vi "CalcPixelShifts.vi"(0 "Sampling Rate (Hz)":dbl=1000000000.0, 1 "c (m/s)":i16=1485, 2 "delay (mm)":sgl, 3 "rf pts":i32, 5 "ROC (m)":dbl=0.012, 9 "Radii (m)":sgl[](array[numeric])=[0.0, 0.00132, 0.00142, 0.0019, 0.002, 0.00236, 0.00245, 0.00275, 0.00285, 0.0031], 11 "One Way Receive":bool, 14 "Dual mode":bool) -> (15 "InterpIndex":sgl[][](array[numeric]))   [LabVIEW 2022 SP3]
panel:
  out "z grid RF samps":dbl[](array[numeric])
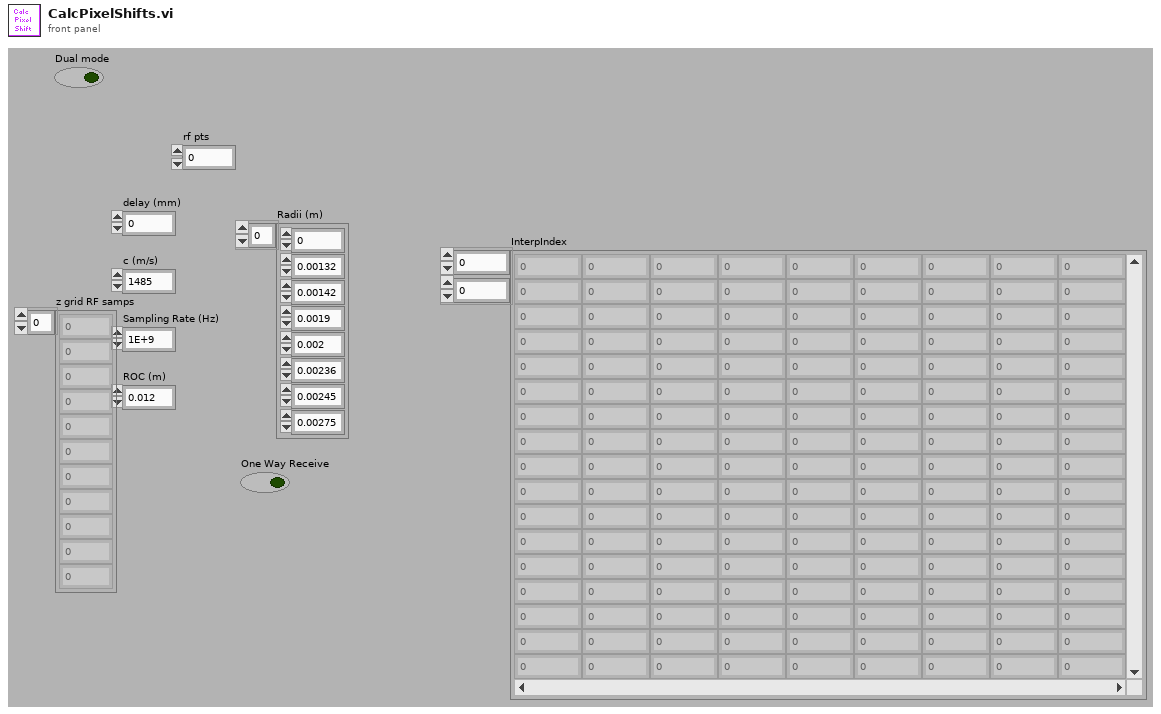
[diagram p1: front panel]
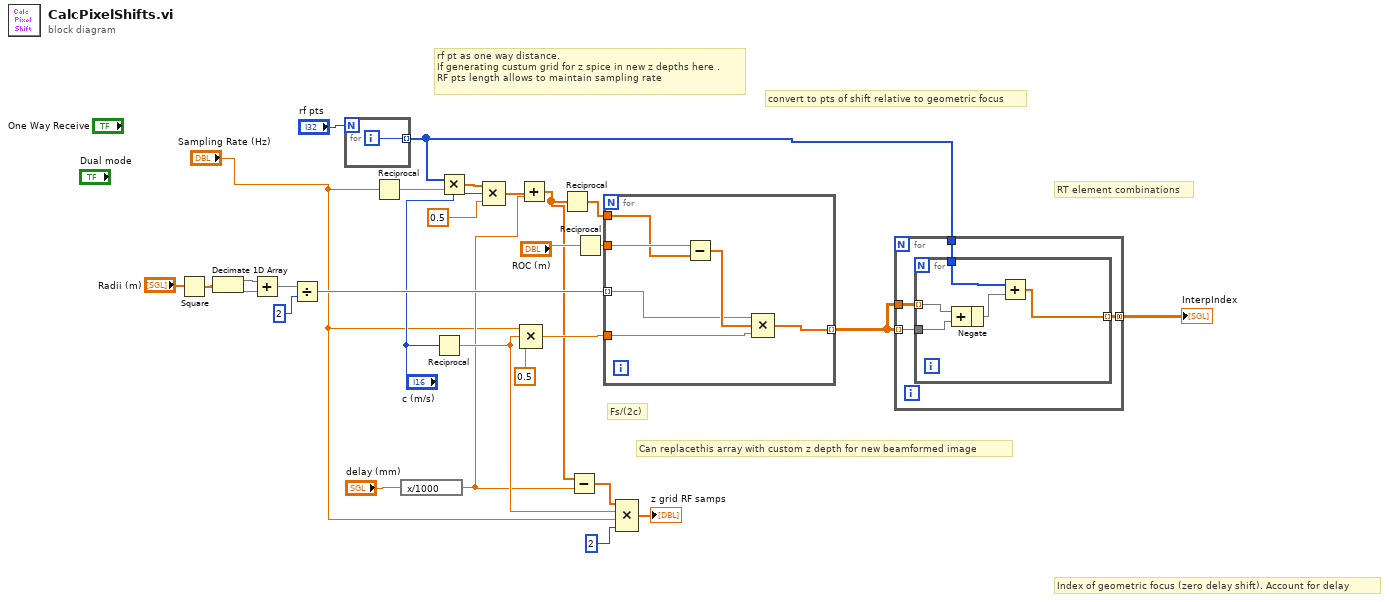
[diagram p0: block diagram]
diagram:
  # "Can replacethis array with custom z depth for new beamformed image"
  # "Index of geometric focus (zero delay shift). Account for delay"
  # "RT element combinations"
  # "convert to pts of shift relative to geometric focus"
  # "rf pt as one way distance.\nIf generating custum grid for z spice in new z depths here .\nRF pts length allows to maintain sampling rate"
  # "Fs/(2c)"
  n1 = Square(x="Radii (m)") -> (x^2=w28:sgl[])
  n2 = Decimate 1D Array(w28) -> (w24:sgl[], w27:sgl[])
  n3 = Add(x=w24, y=w27) -> (x+y=w25:sgl[])
  n4 = Divide(x=w25, y=2) -> (x/y=w23:sgl[])
  n5 = for {
    N: "rf pts" -> [_]
    tunnel: [w30] -> w10 mode=indexing
    i -> [w30]
  }
  n6 = Reciprocal(x="Sampling Rate (Hz)") -> (1/x=w20:dbl)
  n7 = expression code="x/1000"("delay (mm)") -> (w7:sgl)
  n8 = Reciprocal(x="c (m/s)") -> (1/x=w13:dbl)
  n9 = Multiply(x=w10, y=w20) -> (x*y=w12:dbl[])
  n10 = Compound Arithmetic op=MULTIPLY(w12, "c (m/s)", 0.5) -> (w5:dbl[])
  n11 = Add(x=w5, y=w7) -> (x+y=w3:dbl[])
  n12 = Compound Arithmetic op=MULTIPLY("Sampling Rate (Hz)", w13, 0.5) -> (w16:dbl)
  n13 = Reciprocal(x=w3) -> (1/x=w18:dbl[])
  n14 = Subtract(x=w3, y=w7) -> (x-y=w2:dbl[])
  n15 = Reciprocal(x="ROC (m)") -> (1/x=w22:dbl)
  n16 = for {
    tunnel: w23 -> [w34] mode=indexing
    tunnel: w22 -> [w36]
    tunnel: w16 -> [w33]
    tunnel: [w32] -> w19 mode=indexing
    tunnel: w18 -> [w31]
    n17 = Subtract(x=w36, y=w31) -> (x-y=w35:dbl[])
    n18 = Compound Arithmetic op=MULTIPLY(w34, w35, w33) -> (w32:dbl[])
  }
  n19 = Compound Arithmetic op=MULTIPLY(w2, w13, "Sampling Rate (Hz)", 2) -> (→"z grid RF samps":dbl[])
  n20 = for {
    tunnel: w19 -> [w40] mode=indexing
    tunnel: w19 -> [w39]
    tunnel: [w38] -> w6 mode=concatenating
    tunnel: w10 -> [w37]
    n21 = for {
      tunnel: w40 -> [w46]
      tunnel: w39 -> [w45] mode=indexing
      tunnel: [w41] -> w38 mode=indexing
      tunnel: w37 -> [w44]
      n22 = Add(x=w45, y=w46) -> (x+y=w43:dbl[])
      n23 = Negate(x=w43) -> (-x=w42:dbl[])
      n24 = Add(x=w44, y=w42) -> (x+y=w41:dbl[])
    }
  }
  "InterpIndex" <- w6
